vi "Create Listener.vi"(8 "error in (no error)":errorcluster, 10 "Connection Configuration":refnum<class "Connection.lvclass">) -> (0 "error out":errorcluster, 3 "Listener":refnum<class "Connection.lvclass">)   [LabVIEW 2013, in "MQTT_Connection.lvlib" / "Connection.lvclass"]
uses:
  Connection.lvclass
  Connection.lvclass/Connection.ctl
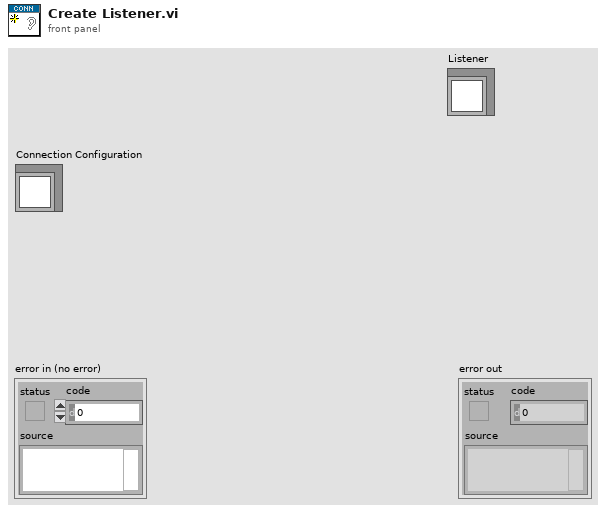
[diagram p1: front panel]
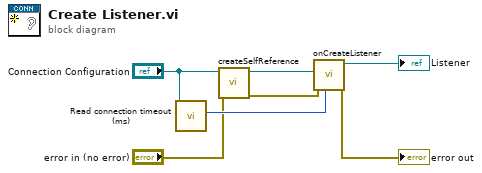
[diagram p0: block diagram]
diagram:
  n1 = call "Read connection timeout (ms).vi"("Connection in"="Connection Configuration") -> ("connection timeout (ms)"=w5:i32)  [unwired: 8 in, 2 out]
  n2 = call "createSelfReference.vi"("error in (no error)"="error in (no error)", "Connection in"="Connection Configuration") -> ("error out"=w1:errorcluster, "Connection out"=w3:refnum<class "Connection.lvclass">)  [unwired: 8 in]
  n3 = call-dynamic "onCreateListener.vi"("timeout (ms)"=w5, "error in (no error)"=w1, "Configuration"=w3) -> ("error out"=→"error out":errorcluster, "Listener"=→"Listener":refnum<class "Connection.lvclass">)  [unwired: 7 in]
